vi "TimeKeeper.vi"() -> ()   [LabVIEW 2015]
uses:
  <vilib>/Platform/TimedLoop/XDataNode/timing_clust.ctl
  <vilib>/Platform/TimedLoop/XDataNode/nitl_modes.ctl
  <vilib>/Platform/TimedLoop/XDataNode/wakeup.ctl
  <vilib>/rvi/Emulation/niFpgaGetClockAttributes.vi
  <vilib>/rvi/Emulation/niFpgaSctlEmulationGetInTimedLoop.vi
  <vilib>/rvi/Emulation/niFpgaEmulationReportErrorSimple.vi
  <vilib>/rvi/Emulation/niFpgaCriticalErrorInLSC.vi
  <vilib>/rvi/Emulation/niFpgaProcessEmulError.vi
  <vilib>/rvi/eio/common/nirviEmuTemplateMethod_errors.vi
  <vilib>/Platform/TimedLoop/XDataNode/XDataNode.xnode
  <vilib>/eio/EIONode/EIONode.xnode
  FPGA Timekeeper.lvlib
  <vilib>/Platform/TimedLoop/XDataNode/XDNodeRunTimeDep.lvlib
  PPS_Global_Var.vi
panel:
  out "FPGA Timekeeper time (ns)":u64
  out "FPGA Timekeeper locked":bool
  out "offset from time reference":i32
  in  "absolute time offset(ns)":u64
  out "PPS":bool
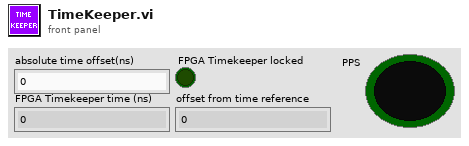
[diagram p1: front panel]
types:
  T1 = typedef "XDNodeRunTimeDep.lvlib/timing_clust.ctl" = cluster{"Expected End [f-1]":u64, "Actual End [f-1]":u64, "Finished Late? [f-1]":bool, "Expected End [i-1]":u64, "Actual End [i-1]":u64, "Finished Late? [i-1]":bool, "Expected Start [i]":u64, "Actual Start [i]":u64, "Expected Start [f]":u64, "Actual Start [f]":u64, "Source Name":string, "Structure Name":string, "Period":i64, "Deadline":i64, "Offset":i64, "Start":i64, "Priority":i32, "Timeout":i32, "Mode":T2, "Wakeup Reason":T3, "Error":errorcluster, "Source Type":string, "Secondary Source Type":string, "Global End Time":u64, "Global Start Time":u64, "Frame Duration":u64, "Iteration Duration":u64, "Assigned CPU":i32, "I/O Scan Engine Mode":u32}
  T2 = typedef "XDNodeRunTimeDep.lvlib/nitl_modes.ctl" = enum32{"No Change", "Process missed periods, maintain original phase", "Discard missed periods, maintain original phase", "Process missed periods, ignore original phase", "Discard missed periods, ignore original phase"}
  T3 = typedef "XDNodeRunTimeDep.lvlib/wakeup.ctl" = enum32{"Normal", "Aborted", "Asynchronous wakeup", "Timing source error", "Timed loop error", "Timeout"}
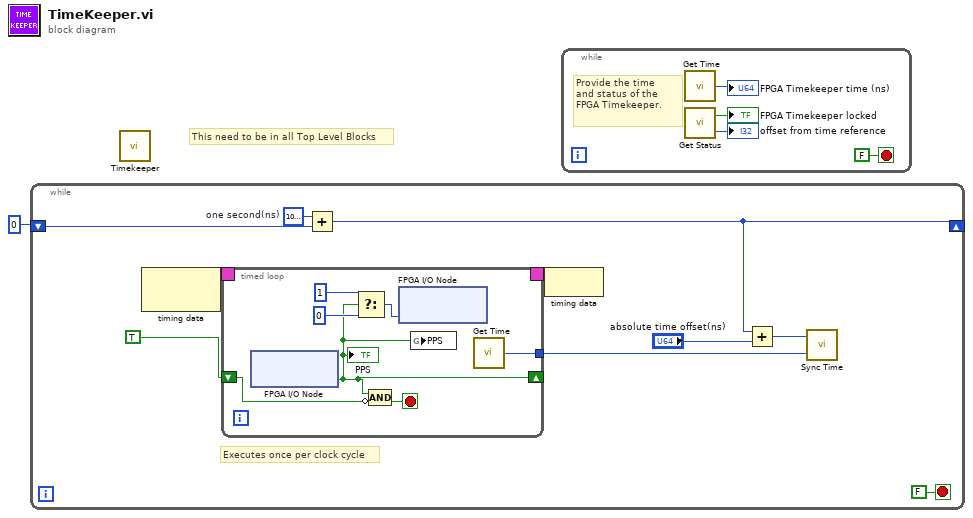
[diagram p0: block diagram]
diagram:
  # "This need to be in all Top Level Blocks"
  n1 = while {
    shift-right: [w4] -> _
    shift-left: u64 0 -> [w11]
    stop <- FALSE stop-if-true
    w10 = u64 1000000000  # one second(ns)
    # "Executes once per clock cycle"
    n2 = node-c288() -> (w9:T1)  [unwired: 1 in]
    n3 = timed-loop {
      timing: w9 -> [_]
      timing-out: [_] -> w8
      shift-right: [w12] -> _
      shift-left: TRUE ("Mod1/DIO0") -> [w18]
      tunnel: [w16] -> w6
      stop <- w17 stop-if-true
      n4 = xnode "FPGA I/O Node"() -> ("GPS PPS"=w12:bool)  [unwired: 1 in, 1 out]
      "PPS" <- w12
      n5 = Select(t=i16 1, s=w12, f=i16 0) -> (s? t:f=w15:i16)
      n6 = Compound Arithmetic op=AND(w12, invert w18) -> (w17:bool)
      n7 = xnode "FPGA I/O Node"("LED/PPS"=w15) -> ()  [unwired: 1 in, 1 out]
      n8 = global write "PPS_Global_Var.vi" "PPS"(w12) -> ()
      n9 = call "Get Time.vi"() -> ("time (ns)"=w16:u64)
    }
    n10 = Add(x=w10, y=w11) -> (x+y=w4:u64)
    n11 = node-c288(w8) -> ()
    n12 = Add(x=w4, y="absolute time offset(ns)") -> (x+y=w3:u64)
    n13 = call "Sync Time.vi"("FPGA Timekeeper time (ns)"=w6, "time reference time (ns)"=w3) -> ()
  }
  n14 = call "Timekeeper.vi"() -> ()  [unwired: 12 in]
  n15 = while {
    stop <- FALSE stop-if-true
    # "Provide the time\nand status of the\nFPGA Timekeeper."
    n16 = call "Get Time.vi"() -> ("time (ns)"=→"FPGA Timekeeper time (ns)":u64)
    n17 = call "Get Status.vi"() -> ("FPGA Timekeeper locked"=→"FPGA Timekeeper locked":bool, "offset from time reference"=→"offset from time reference":i32)
  }
